vi "From String.vi"(8 "error in (no error)":errorcluster, 9 "initial scan location":u32, 10 "String":string, 11 "Type in":refnum<class "Abs_String 1D.lvclass">) -> (0 "error out":errorcluster, 1 "offset past scan":u32, 2 "Remaining String":string, 3 "Type out":refnum<class "Abs_String 1D.lvclass">)   [LabVIEW 2021, in "Abs_String 1D.lvclass"]
uses:
  Abs_String 1D.lvclass
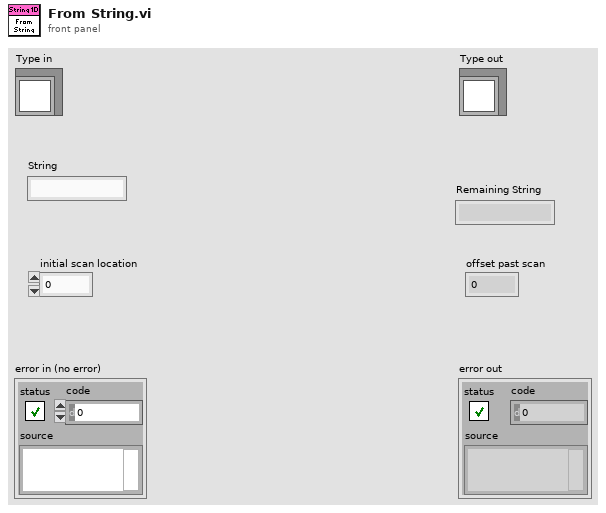
[diagram p1: front panel]
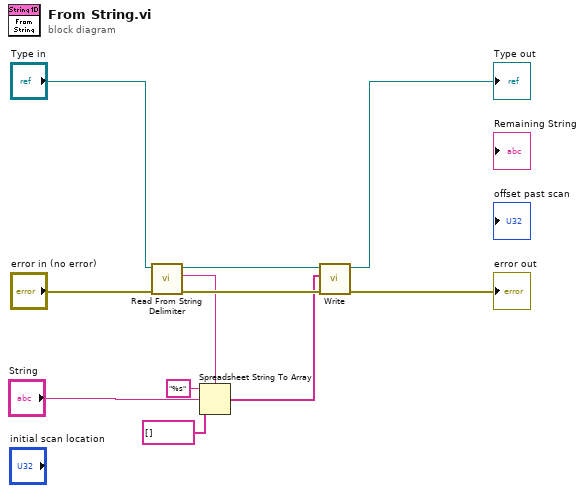
[diagram p0: block diagram]
diagram:
  n1 = call-dynamic "Read From String Delimiter.vi"("error in (no error)"="error in (no error)", "Abs_Array in"="Type in") -> ("error out"=w8:errorcluster, "From String Delimiter"=w5:string, "Abs_Array out"=w6:refnum<class "Abs_String 1D.lvclass">)  [unwired: 7 in]
  n2 = Spreadsheet String To Array(delimiter (Tab)=w5, format string="%s", spreadsheet string="String", array type (2D Dbl)=string[] []) -> (array=w1:string[])
  n3 = call-dynamic "Write.vi"("error in (no error)"=w8, "Array"=w1, "Abs_String in"=w6) -> ("error out"=→"error out":errorcluster, "Abs_String out"=→"Type out":refnum<class "Abs_String 1D.lvclass">)  [unwired: 7 in]
